vi "valves_flushprogram.vi"(0 "Input solution":dbl=1.0, 1 "COM4 in":refnum<k24>, 2 "Add to C":dbl, 3 "Rings to open":u32, 4 "Cycles":i32=1, 5 "error in":errorcluster) -> (6 "COM4 out":refnum<k24>, 7 "error out":errorcluster)   [LabVIEW 2018]
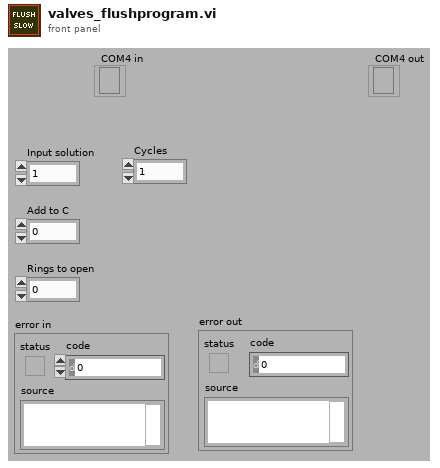
[diagram p1: front panel]
types:
  T1 = cluster{"Op A":u8[], "Op B":u8[], "Op C":u8[], "open":u8[], "L 3 A":u8[], "L 4 A 16":u8[], "F1 A":u8[], "L 4 A 34":u8[], "L 4 A 5":u8[], "FPw1 A":u8[], "L 2 A":u8[], "L 1 C FS":u8[], "L 2 C FS":u8[], "L 4 C 456 FS":u8[], "L 4 C 123 FS":u8[], "L 1 A":u8[], "L 1 C":u8[], "L 2 C":u8[], "L 4 C 456":u8[], "L 4 C 123":u8[], "FPw1 C":u8[], "F1 B":u8[], "F1 C":u8[], "F2 C":u8[], "F5 C":u8[]}
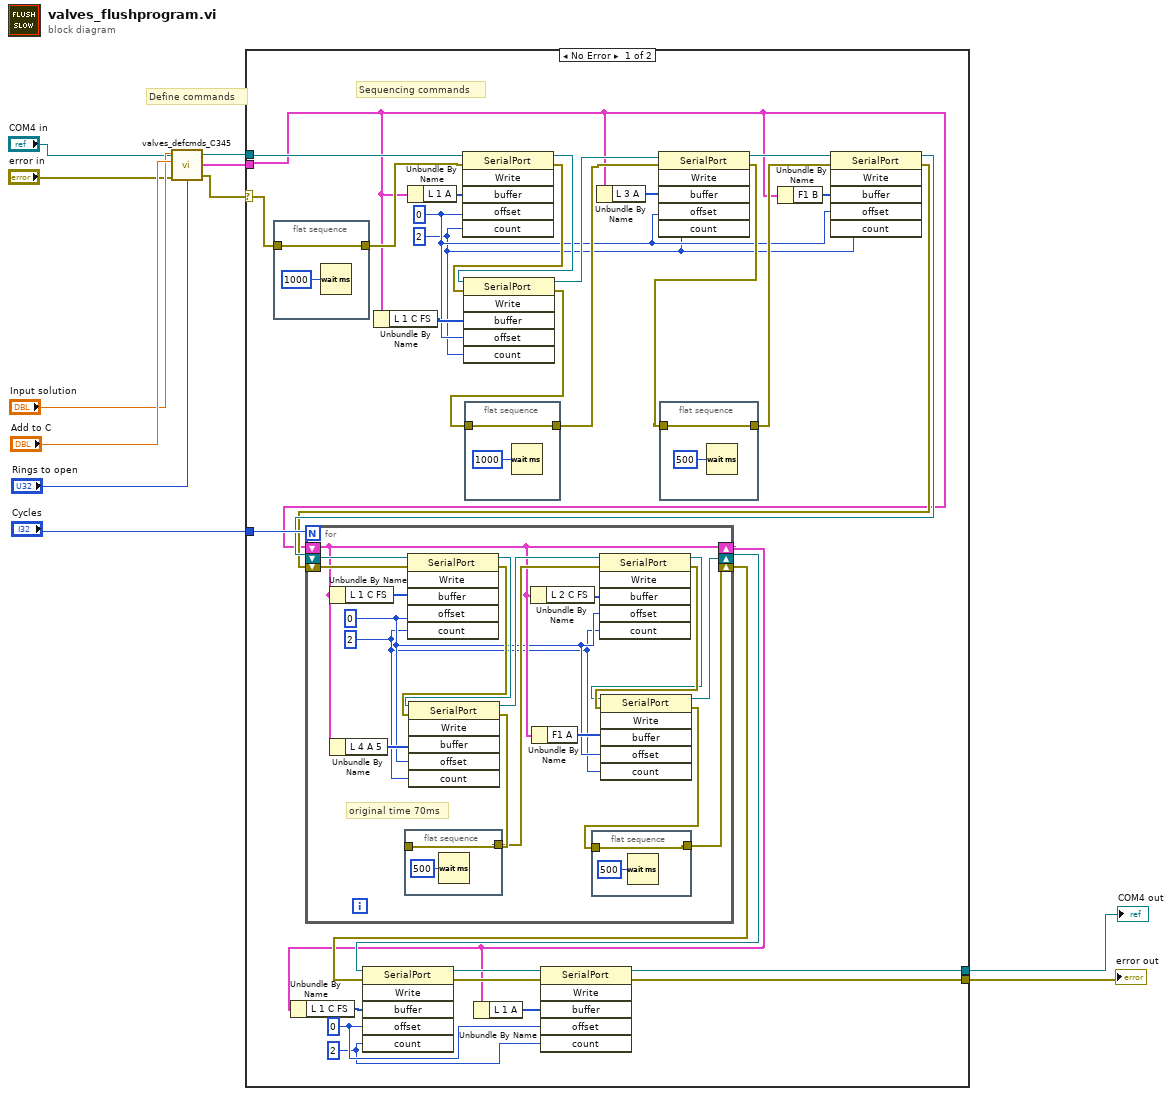
[diagram p0: block diagram]
diagram:
  # "Define commands"
  n1 = call "valves_defcmds_C345.vi"("Input solution"="Input solution", "Add to C"="Add to C", "Rings to open"="Rings to open", "error in"="error in", "COM4 in"="COM4 in") -> ("COM4 out"=w8:refnum<k24>, "Commands out"=w10:T1, "error out"=w11:errorcluster)
  n2 = case shown="No Error" w11 {
    selector: w11 -> [w29 w74]
    tunnel: "Cycles" -> [w43 _]
    tunnel: w8 -> [w30 w73]
    tunnel: [w24 w74] -> w3
    tunnel: [w23 w73] -> w1
    tunnel: w10 -> [w26 _]
    frame No Error {
      w12 = 2 ("count")
      w13 = 0 ("offset")
      w14 = 2 ("count")
      w15 = 0 ("offset")
      # "Sequencing commands"
      n3 = flat-sequence {
        tunnel: [w71] -> w42
        tunnel: w29 -> [w71]
        frame #0 {
          n4 = Wait (ms)(milliseconds to wait=u32 1000) -> ()  [unwired: 1 out]
        }
      }
      n5 = Unbundle By Name(w26) -> ("L 1 C FS"=w20:u8[])
      n6 = Unbundle By Name(w26) -> ("L 1 A"=w21:u8[])
      n7 = invoke class="SerialPort" method="Write"(reference=w30, error in=w42, "buffer"=w21, "offset"=w15, "count"=w14) -> (reference out=w39:refnum<k24>, error out=w41:errorcluster)  [unwired: 1 in, 4 out]
      n8 = invoke class="SerialPort" method="Write"(reference=w39, error in=w41, "buffer"=w20, "offset"=w15, "count"=w14) -> (reference out=w27:refnum<k24>, error out=w40:errorcluster)  [unwired: 1 in, 4 out]
      n9 = flat-sequence {
        tunnel: [w69] -> w28
        tunnel: w40 -> [w69]
        frame #0 {
          n10 = Wait (ms)(milliseconds to wait=u32 1000) -> ()  [unwired: 1 out]
        }
      }
      n11 = Unbundle By Name(w26) -> ("L 3 A"=w19:u8[])
      n12 = invoke class="SerialPort" method="Write"(reference=w27, error in=w28, "buffer"=w19, "offset"=w15, "count"=w14) -> (reference out=w36:refnum<k24>, error out=w38:errorcluster)  [unwired: 1 in, 4 out]
      n13 = flat-sequence {
        tunnel: [w67] -> w37
        tunnel: w38 -> [w67]
        frame #0 {
          n14 = Wait (ms)(milliseconds to wait=u32 500) -> ()  [unwired: 1 out]
        }
      }
      n15 = Unbundle By Name(w26) -> ("F1 B"=w18:u8[])
      n16 = invoke class="SerialPort" method="Write"(reference=w36, error in=w37, "buffer"=w18, "offset"=w15, "count"=w14) -> (reference out=w35:refnum<k24>, error out=w34:errorcluster)  [unwired: 1 in, 4 out]
      n17 = for {
        N: w43 -> [_]
        shift-right: [w50] -> w25
        shift-left: w34 -> [w59]
        shift-right: [w51] -> w31
        shift-left: w35 -> [w62]
        shift-right: [w52] -> w22
        shift-left: w26 -> [w52]
        w44 = 2 ("count")
        w45 = 0 ("offset")
        # "original time 70ms"
        n18 = Unbundle By Name(w52) -> ("L 1 C FS"=w47:u8[])
        n19 = Unbundle By Name(w52) -> ("L 4 A 5"=w46:u8[])
        n20 = flat-sequence {
          tunnel: [w66] -> w56
          tunnel: w57 -> [w66]
          frame #0 {
            n21 = Wait (ms)(milliseconds to wait=u32 500) -> ()  [unwired: 1 out]
          }
        }
        n22 = invoke class="SerialPort" method="Write"(reference=w62, error in=w59, "buffer"=w47, "offset"=w45, "count"=w44) -> (reference out=w61:refnum<k24>, error out=w58:errorcluster)  [unwired: 1 in, 4 out]
        n23 = invoke class="SerialPort" method="Write"(reference=w61, error in=w58, "buffer"=w46, "offset"=w45, "count"=w44) -> (reference out=w60:refnum<k24>, error out=w57:errorcluster)  [unwired: 1 in, 4 out]
        n24 = Unbundle By Name(w52) -> ("L 2 C FS"=w48:u8[])
        n25 = Unbundle By Name(w52) -> ("F1 A"=w49:u8[])
        n26 = flat-sequence {
          tunnel: w53 -> [w64]
          tunnel: [w64] -> w50
          frame #0 {
            n27 = Wait (ms)(milliseconds to wait=u32 500) -> ()  [unwired: 1 out]
          }
        }
        n28 = invoke class="SerialPort" method="Write"(reference=w60, error in=w56, "buffer"=w48, "offset"=w45, "count"=w44) -> (reference out=w54:refnum<k24>, error out=w55:errorcluster)  [unwired: 1 in, 4 out]
        n29 = invoke class="SerialPort" method="Write"(reference=w54, error in=w55, "buffer"=w49, "offset"=w45, "count"=w44) -> (reference out=w51:refnum<k24>, error out=w53:errorcluster)  [unwired: 1 in, 4 out]
      }
      n30 = Unbundle By Name(w22) -> ("L 1 C FS"=w16:u8[])
      n31 = invoke class="SerialPort" method="Write"(reference=w31, error in=w25, "buffer"=w16, "offset"=w13, "count"=w12) -> (reference out=w32:refnum<k24>, error out=w33:errorcluster)  [unwired: 1 in, 4 out]
      n32 = Unbundle By Name(w22) -> ("L 1 A"=w17:u8[])
      n33 = invoke class="SerialPort" method="Write"(reference=w32, error in=w33, "buffer"=w17, "offset"=w13, "count"=w12) -> (reference out=w23:refnum<k24>, error out=w24:errorcluster)  [unwired: 1 in, 4 out]
    }
    frame Error {
    }
  }
  "error out" <- w3
  "COM4 out" <- w1
